vi "multiplier32.vi"(1 "Y":i32, 2 "X":i32) -> (0 "XY":i32)   [LabVIEW 2009]
doc: "Multiplies two I32's. Output is an I32."
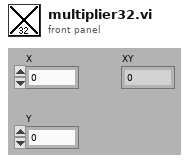
[diagram p1: front panel]
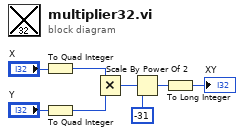
[diagram p0: block diagram]
diagram:
  n1 = To Quad Integer(1:"X") -> (0:w4:i64)
  n2 = To Quad Integer(1:"Y") -> (0:w2:i64)
  n3 = Multiply(x=w4, y=w2) -> (x*y=w8:i64)
  n4 = Scale By Power Of 2(n=i16 -31, x=w8) -> (x*2^n=w6:i64)
  n5 = To Long Integer(number=w6) -> (32bit integer=→"XY":i32)
